vi "DQMH Load Module.vi"(7 "Module Disk Path":path, 8 "error in (no error)":errorcluster, 11 "Application reference":refnum<vi>) -> (0 "error out":errorcluster)   [LabVIEW 2022 SP3, in "hse-dqmh-dynamicrequesters.lvlib"]
doc: "Calls the \"Load Module\" request VI of the module in <b>path</b>\n\n____\nHAMPEL SOFTWARE ENGINEERING v3.8.0 (2023-12-18 14:41)"
uses:
  hse-dqmh-dynamicrequesters.lvlib
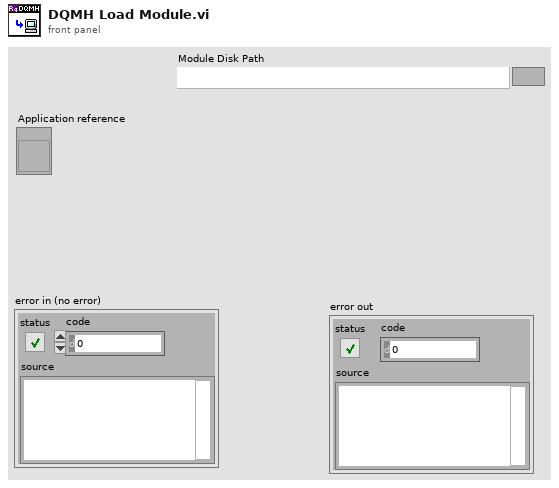
[diagram p1: front panel]
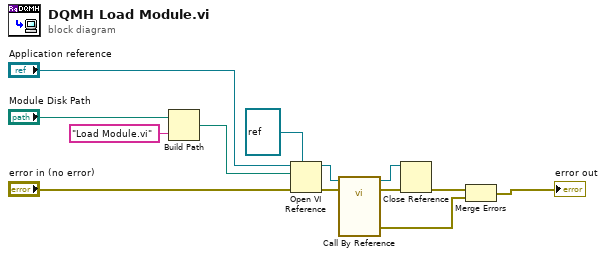
[diagram p0: block diagram]
diagram:
  n1 = Build Path(base path="Module Disk Path", name or relative path="Load Module.vi") -> (appended path=w2:path)
  n2 = Open VI Reference(type specifier VI Refnum (for type only)=refnum<vi> refnum, application reference (local)="Application reference", vi path=w2, error in (no error)="error in (no error)") -> (vi reference=w3:refnum<vi>, error out=w4:errorcluster)  [unwired: 2 in]
  n3 = call-by-ref "?"(reference=w3, error in=w4) -> (reference out=w9:refnum<vi>, error out=w8:errorcluster, 0:"error out"=w11:errorcluster)  [unwired: 11 in]
  n4 = Close Reference(reference=w9, error in (no error)=w8) -> (error out=w7:errorcluster)
  n5 = Merge Errors(w7, w11) -> (→"error out":errorcluster)
